vi "Pane Size.vi"(8 "error in (no error)":errorcluster, 11 "2DArrayManager in":refnum<class "2DArrayManager.lvclass">) -> (0 "error out":errorcluster, 3 "2DArrayManager out":refnum<class "2DArrayManager.lvclass">)   [LabVIEW 2020, in "OOPanel.lvlib" / "2DArrayManager.lvclass"]
uses:
  2DArrayManager.lvclass
  2DArrayManager.lvclass/2DArrayManager.ctl
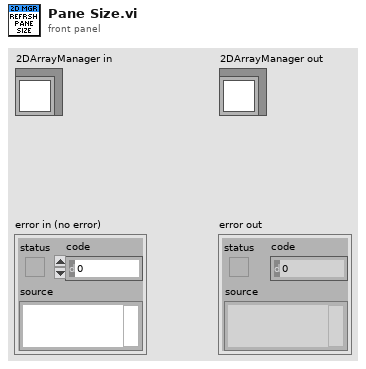
[diagram p1: front panel]
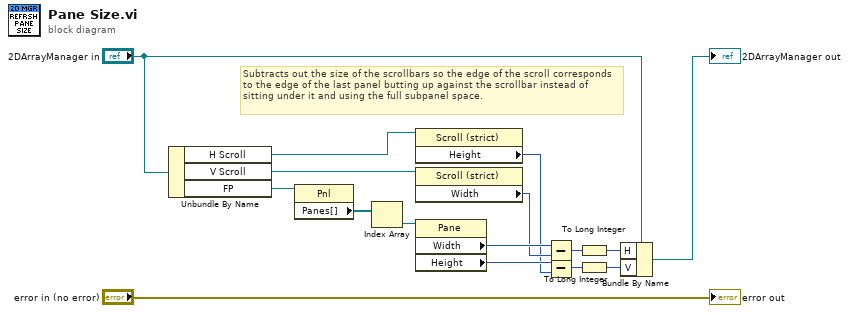
[diagram p0: block diagram]
diagram:
  # "Subtracts out the size of the scrollbars so the edge of the scroll corresponds to the edge of the last panel butting up against the scrollbar instead of sitting under it and using the full subpanel space."
  n1 = Unbundle By Name("2DArrayManager in") -> ("H Scroll"=w5:refnum<vi>, "V Scroll"=w6:refnum<vi>, "FP"=w12:refnum<vi>)
  n2 = property class="Pnl"(reference=w12) -> ("Panes[]"=w14:refnum<vi>[])  [unwired: 1 in, 2 out]
  n3 = Index Array(array=w14) -> (element=w13:refnum<vi>)  [unwired: 1 in]
  n4 = property class="Scroll (strict)"(reference=w5) -> ("Height"=w1:u32)  [unwired: 1 in, 2 out]
  n5 = property class="Scroll (strict)"(reference=w6) -> ("Width"=w2:u32)  [unwired: 1 in, 2 out]
  n6 = property class="Pane"(reference=w13) -> ("Width"=w10:u32, "Height"=w9:u32)  [unwired: 1 in, 2 out]
  n7 = Subtract(x=w10, y=w2) -> (x-y=w4:u32)
  n8 = Subtract(x=w9, y=w1) -> (x-y=w3:u32)
  n9 = To Long Integer(number=w4) -> (32bit integer=w8:i32)
  n10 = To Long Integer(number=w3) -> (32bit integer=w7:i32)
  n11 = Bundle By Name(cluster="2DArrayManager in", "H"=w8, "V"=w7) -> (→"2DArrayManager out":refnum<class "2DArrayManager.lvclass">)
  "error out" <- "error in (no error)"
